vi "Sound.vi"() -> ()   [LabVIEW 2019]
uses:
  <vilib>/Analysis/5stat.llb/RMS (DBL).vi
  <vilib>/measure/mascope.llb/Amplitude and Levels N chan.vi
  <vilib>/Analysis/NI_AALPro.lvlib
  <vilib>/measure/NI_MAPro.lvlib
panel:
  out "Zero Crossing":dbl
  out "Roll up":dbl
  out "Centroid":dbl
  out "BPM":dbl
  in  "Channel":dbl
  in  "Sample value":dbl
  out "RMS":dbl format="%0.2f"
  out "data":waveform(dbl)[](array[waveform])
  out "Waveform Graph":waveform(dbl)[](graph)
  in  "path":path
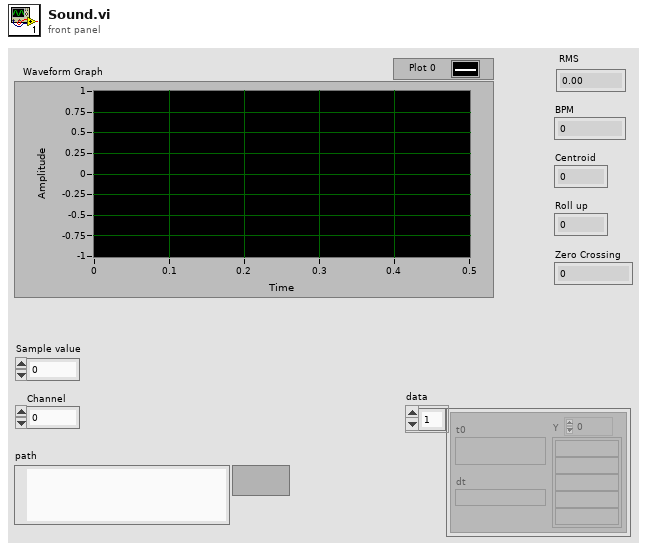
[diagram p1: front panel]
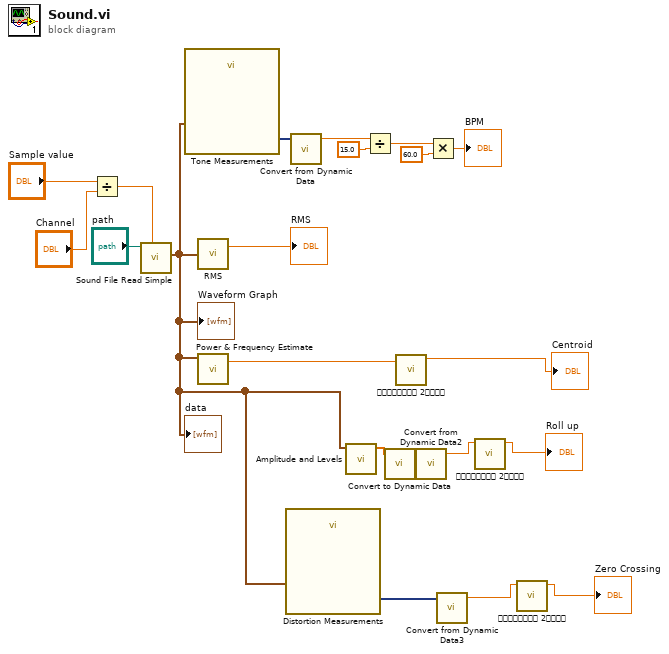
[diagram p0: block diagram]
diagram:
  n1 = Divide(x="Sample value", y="Channel") -> (x/y=w17:dbl)
  n2 = call <vilib>:"Sound File Read Simple.vi"("number of samples/ch (-1: all)"=w17, "path"="path") -> ("data"=w6:waveform(dbl)[])  [unwired: 6 in, 3 out]
  "Waveform Graph" <- w6
  "data" <- w6
  n3 = call "Tone Measurements"("Signals"=w6) -> ("Frequency"=w16:dynamicdata)  [unwired: 9 in, 1 out]
  n4 = call-poly <vilib>:"RMS.vi"("X"=w6) -> ("rms value"=→"RMS":dbl)  [unwired: 1 out]
  n5 = call <vilib>:"Power & Frequency Estimate.vi"("Power Spectrum (V^2 rms)"=w6) -> ("est frequency peak"=w10:dbl)  [unwired: 5 in, 1 out]
  n6 = call "Distortion Measurements"("Signals"=w6) -> ("SINAD (dB)"=w5:dynamicdata)  [unwired: 9 in, 1 out]
  n7 = call "Convert from Dynamic Data"("Dynamic Data Type"=w16) -> ("Scalar"=w15:dbl)  [unwired: 3 in]
  n8 = call-poly <vilib>:"Amplitude and Levels.vi"("signal(s) in"=w6) -> ("amplitude"=w8:dbl[])  [unwired: 7 in, 3 out]
  n9 = Divide(x=w15, y=15.0) -> (x/y=w13:dbl)
  n10 = call "Convert to Dynamic Data"("Array"=w8) -> ("Dynamic Data Type"=w7:dynamicdata)  [unwired: 3 in]
  n11 = call "소숫점 2자리.vi"("input Value"=w10) -> ("output value"=→"Centroid":dbl)  [unwired: 10 in]
  n12 = call "Convert from Dynamic Data2"("Dynamic Data Type"=w7) -> ("Scalar"=w2:dbl)  [unwired: 3 in]
  n13 = Multiply(x=w13, y=60.0) -> (x*y=→"BPM":dbl)
  n14 = call "Convert from Dynamic Data3"("Dynamic Data Type"=w5) -> ("Scalar"=w4:dbl)  [unwired: 3 in]
  n15 = call "소숫점 2자리.vi"("input Value"=w2) -> ("output value"=→"Roll up":dbl)  [unwired: 10 in]
  n16 = call "소숫점 2자리.vi"("input Value"=w4) -> ("output value"=→"Zero Crossing":dbl)  [unwired: 10 in]
